vi "PH_Beckhoff_PP_PU.declare analog InputTags.vi"(3 "PU Type":T3) -> (0 "Analog Inputs":T4, 1 "Description":string)   [LabVIEW 2014, in "PH_Beckhoff_PP_PU.lvlib"]
uses:
  PH_Beckhoff_PP_PU.lvlib
  PH_Beckhoff/PH_Beckhoff.Analog Inputs.ctl
  PH_Beckhoff/PH_Beckhoff.Scaling Type.ctl
  PH_Beckhoff_PP_PU.PU Rack Type.ctl
  PH_PP_Common/PH_PP_Common.PSU Tags.ctl
  PH_Beckhoff/PH_Beckhoff.lvlib
  PH_PP_Common/PH_PP_Common.lvlib
panel:
  in  "Analog Input Value":T2
  out "Right Size?":bool
  # "Let this VI run to check the size!"
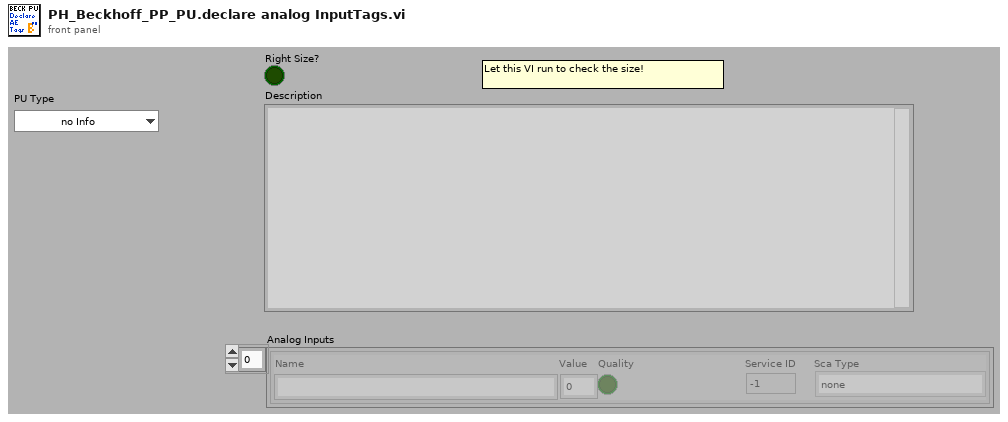
[diagram p1: front panel]
types:
  T1 = typedef "PH_Beckhoff.lvlib/PH_Beckhoff.Scaling Type.ctl" = enum16{"none", "0 ... 15 Bit -> 0 ... 5", "0 ... 15 Bit -> 0 ... 10", "0 ... 15 Bit -> 0 ... 25", "0 ... 15 Bit -> 4 ... 20", "0 ... 15 Bit -> 0 ... 1", "0 ... 15 Bit -> 0 ... 20000", "0 ... 15 Bit -> 0 ... 24000"}
  T2 = cluster{"Name":string, "Value":u32, "Quality":bool, "Service ID":i32, "Sca Type":T1}
  T3 = typedef "PH_Beckhoff_PP_PU.lvlib/PH_Beckhoff_PP_PU.PU Rack Type.ctl" = enum16{"no Info", "PA 19mm", "PA 45mm", "MA PU 1 and 2", "MA PU 3 and 4", "MA PU 5 and 6", "MA FR and PILC"}
  T4 = typedef "PH_Beckhoff.lvlib/PH_Beckhoff.Analog Inputs.ctl" = cluster{"Name":string, "Value":u32, "Quality":bool, "Service ID":i32, "Sca Type":T1}[]
  T5 = typedef "PH_PP_Common.lvlib/PH_PP_Common.PSU Tags.ctl" = enum16{"voltage-indicator", "peak-detect", "current", "voltage", "inihibit-indicator", "end-of-charge", "HV-on-indicator", "overtemperature", "interlock-indicator", "load-fault", "sum-fault", "HV-off-indicator", "DC-ok", "inhibit", "HV-on", "interlock", "reset", "Status", "Limits"}
  T6 = typedef "PH_PP_Common.lvlib/PH_PP_Common.PUs.ctl" = enum16{"no Info", "PA-19mm-1", "PA-19mm-2", "PA-45mm-PILC", "PA-45mm-MAIN", "MA-PU-1", "MA-PU-2", "MA-PU-3", "MA-PU-4", "MA-PU-5", "MA-PU-6", "MA-FR", "MA-PILC", "PA-45mm-DP"}
  T7 = typedef "PH_PP_Common.lvlib/PH_PP_Common.PSU Type.ctl" = enum16{"none", "Maxwell Standard", "DEL", "Maxwell ALE", "Continuum 601k"}
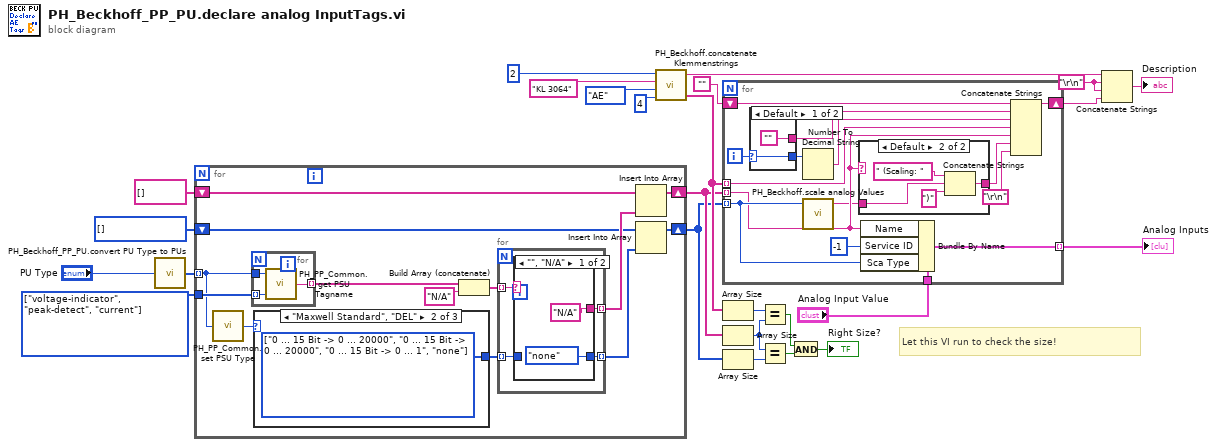
[diagram p0: block diagram]
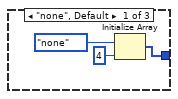
[diagram p2: hidden frame]
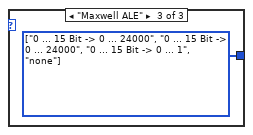
[diagram p3: hidden frame]
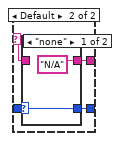
[diagram p4: hidden frame]
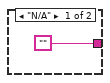
[diagram p6: hidden frame]
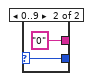
[diagram p7: hidden frame]
diagram:
  w1 = T5[] [enum."voltage-indicator", enum."peak-detect", enum."current"] items=["voltage-indicator", "peak-detect", "current", "voltage", "inihibit-indicator", "end-of-charge", "HV-on-indicator", "overtemperature", "interlock-indicator", "load-fault", "sum-fault", "HV-off-indicator", "DC-ok", "inhibit", "HV-on", "interlock", "reset", "Status", "Limits"]
  w6 = T1[] [] items=["none", "0 ... 15 Bit -> 0 ... 5", "0 ... 15 Bit -> 0 ... 10", "0 ... 15 Bit -> 0 ... 25", "0 ... 15 Bit -> 4 ... 20", "0 ... 15 Bit -> 0 ... 1", "0 ... 15 Bit -> 0 ... 20000", "0 ... 15 Bit -> 0 ... 24000"]
  w23 = "\r\n"
  # "Let this VI run to check the size!"
  n1 = call "PH_Beckhoff_PP_PU.convert PU Type to PUs.vi"("PU Type"="PU Type") -> ("PUs"=w2:T6[])
  n2 = for {
    shift-right: [w37] -> w5
    shift-left: string[] [] -> [w36]
    shift-right: [w35] -> w4
    shift-left: w6 -> [w34]
    tunnel: w2 -> [w27] mode=indexing
    tunnel: w1 -> [w30]
    n3 = call "PH_PP_Common.set PSU Type.vi"("PU"=w27) -> ("PSU Type"=w26:T7)
    n4 = for {
      tunnel: w27 -> [w41]
      tunnel: w30 -> [w40] mode=indexing
      tunnel: [w39] -> w29 mode=indexing
      n5 = call "PH_PP_Common.get PSU Tagname.vi"("PSU Tag"=w40, "PU"=w41) -> ("PSU Tagname"=w39:string)  [unwired: 1 in]
    }
    n6 = case shown="\"Maxwell Standard\", \"DEL\"" w26 {
      tunnel: [w43 w45 w46] -> w33
      frame "none", Default {
        n7 = Initialize Array(PH_Beckhoff.Scaling_Type."none" ("Sca Type"), 4 ("dimension size")) -> (w43:T1[])
      }
      frame "Maxwell Standard", "DEL" {
        w45 = T1[] [enum."0 ... 15 Bit -> 0 ... 20000", enum."0 ... 15 Bit -> 0 ... 20000", enum."0 ... 15 Bit -> 0 ... 1", enum."none"] items=["none", "0 ... 15 Bit -> 0 ... 5", "0 ... 15 Bit -> 0 ... 10", "0 ... 15 Bit -> 0 ... 25", "0 ... 15 Bit -> 4 ... 20", "0 ... 15 Bit -> 0 ... 1", "0 ... 15 Bit -> 0 ... 20000", "0 ... 15 Bit -> 0 ... 24000"]
      }
      frame "Maxwell ALE" {
        w46 = T1[] [enum."0 ... 15 Bit -> 0 ... 24000", enum."0 ... 15 Bit -> 0 ... 24000", enum."0 ... 15 Bit -> 0 ... 1", enum."none"] items=["none", "0 ... 15 Bit -> 0 ... 5", "0 ... 15 Bit -> 0 ... 10", "0 ... 15 Bit -> 0 ... 25", "0 ... 15 Bit -> 4 ... 20", "0 ... 15 Bit -> 0 ... 1", "0 ... 15 Bit -> 0 ... 20000", "0 ... 15 Bit -> 0 ... 24000"]
      }
    }
    n8 = Build Array (concatenate)(w29, "N/A" ("t")) -> (w31:string[])
    n9 = for {
      tunnel: w31 -> [w49] mode=indexing
      tunnel: w33 -> [w48] mode=indexing
      tunnel: [w50] -> w38 mode=indexing
      tunnel: [w47] -> w32 mode=indexing
      n10 = case shown="\"\", \"N/A\"" w49 {
        selector: w49 -> [_ w55]
        tunnel: ["N/A" w56] -> w50
        tunnel: w48 -> [_ w54]
        tunnel: [PH_Beckhoff.Scaling_Type."none" ("Sca Type") w53] -> w47
        frame "", "N/A" {
        }
        frame Default {
          n11 = case shown="\"none\"" w54 {
            selector: w54 -> [w57 w60]
            tunnel: ["N/A" w59] -> w56
            tunnel: w55 -> [_ w59]
            tunnel: [w57 w60] -> w53
            frame "none" {
            }
            frame Default {
            }
          }
        }
      }
    }
    n12 = Insert Into Array(array=w36, new element=w38) -> (w37:string[])  [unwired: 1 in]
    n13 = Insert Into Array(array=w34, new element=w32) -> (w35:T1[])  [unwired: 1 in]
  }
  n14 = call "PH_Beckhoff.concatenate Klemmenstrings.vi"("# of In- or Outputs"=4, "Type"=enum16{"AE", "AA", "DE", "DA", "SE"}."AE", "Klemmenname"="KL 3064", "Quantity"=2) -> ("concatenated string array"=w11:string[], "\"<Type>: <Quantity> x <Klemmenname>\""=w12:string)  [unwired: 1 out]
  n15 = for {
    tunnel: w5 -> [w66] mode=indexing
    tunnel: w11 -> [w71] mode=indexing
    shift-right: [w61] -> w24
    shift-left: "" -> [w62]
    tunnel: w4 -> [w69] mode=indexing
    tunnel: "Analog Input Value" -> [w67]
    tunnel: [w70] -> w10 mode=indexing
    i -> [w75]
    n16 = case shown="Default" w75 {
      selector: w75 -> [w81 w84]
      tunnel: [w81 w84] -> w74
      tunnel: ["" "0"] -> w73
      frame Default {
      }
      frame 0..9 {
      }
    }
    n17 = Number To Decimal String(number=w74) -> (decimal integer string=w72:string)  [unwired: 1 in]
    n18 = call "PH_Beckhoff.scale analog Values.vi"("Sca Type"=w69) -> ("Scaling"=w65:string)  [unwired: 2 in, 2 out]
    n19 = case shown="Default" w66 {
      tunnel: w65 -> [_ w79]
      tunnel: ["" w77] -> w64
      frame "N/A" {
      }
      frame Default {
        n20 = Concatenate Strings(" (Scaling: " ("string"), w79, ")" ("string")) -> (w77:string)
      }
    }
    n21 = Bundle By Name(cluster=w67, "Name"=w66, "Service ID"=-1, "Sca Type"=w69) -> (w70:T2)
    n22 = Concatenate Strings(w62, w73, w72, w71, w66, w64, "\r\n") -> (w61:string)
  }
  "Analog Inputs" <- w10
  n23 = Array Size(array=w11) -> (size(s)=w21:i32)
  n24 = Array Size(array=w5) -> (size(s)=w17:i32)
  n25 = Array Size(array=w4) -> (size(s)=w16:i32)
  n26 = Equal?(x=w21, y=w17) -> (x = y?=w20:bool)
  n27 = Equal?(x=w17, y=w16) -> (x = y?=w14:bool)
  n28 = And(x=w20, y=w14) -> (x .and. y?=→"Right Size?":bool)
  n29 = Concatenate Strings(w12, w23, w23, w24) -> (→"Description":string)
